vi "Boolean.vi"() -> ()   [LabVIEW 2019]
panel:
  out "Boolean 2":bool
  in  "Boolean":bool
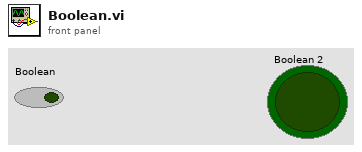
[diagram p1: front panel]
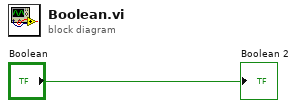
[diagram p0: block diagram]
diagram:
  "Boolean 2" <- "Boolean"
